vi "4_9.vi"() -> ()   [LabVIEW 2020]
panel:
  out "Output":string
  in  "Input":string
  out "substring":string
  out "Array":string[](array[string])
  in  "string":string
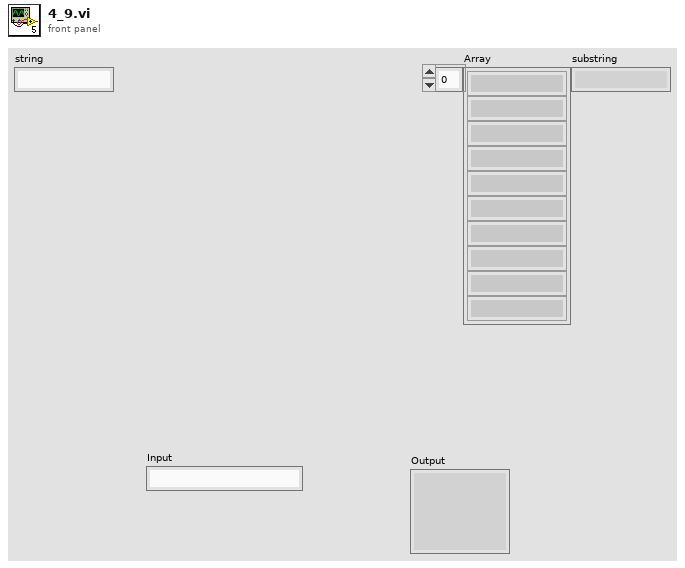
[diagram p1: front panel]
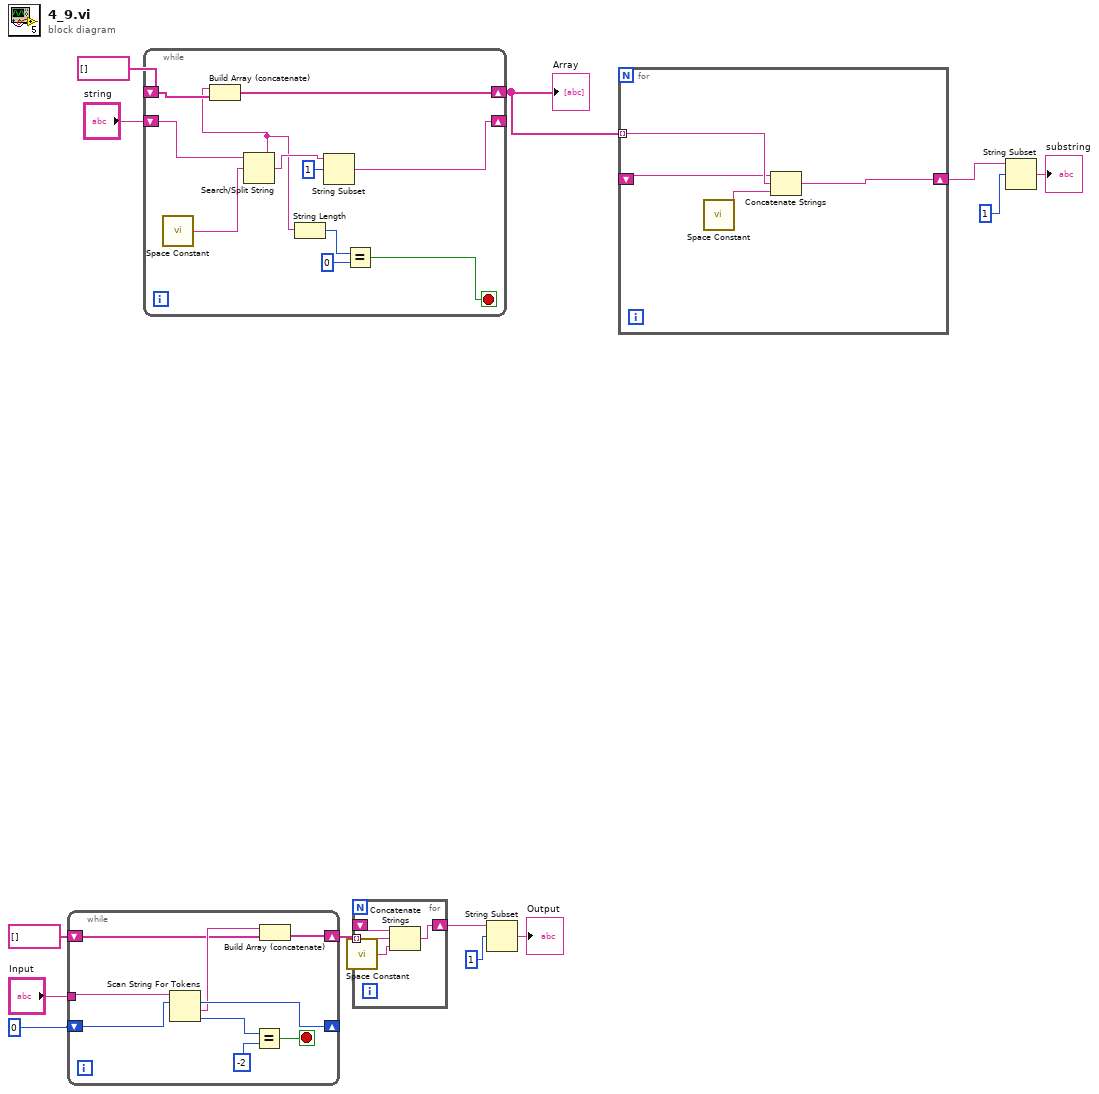
[diagram p0: block diagram]
diagram:
  n1 = while {
    tunnel: "Input" -> [w22]
    shift-right: [w18] -> w5
    shift-left: string[] [] -> [w14]
    shift-right: [w17] -> _
    shift-left: 0 ("offset past token") -> [w16]
    stop <- w19 stop-if-true
    n2 = Scan String For Tokens(8:w16, 9:w22) -> (0:w21:i32, 1:w15:string, 2:w17:i32)  [unwired: 4 in, 1 out]
    n3 = Equal?(x=w21, y=-2) -> (x = y?=w19:bool)
    n4 = Build Array (concatenate)(w15, w14) -> (w18:string[])
  }
  n5 = while {
    shift-right: [w29] -> _
    shift-left: "string" -> [w33]
    shift-right: [w28] -> w11
    shift-left: string[] [] -> [w24]
    stop <- w25 stop-if-true
    n6 = call <vilib>:"Space Constant.vi"() -> ("String"=w32:string)
    n7 = Search/Split String(string=w33, search string/char (-)=w32) -> (substring before match=w23:string, match + rest of string=w30:string)  [unwired: 1 in, 1 out]
    n8 = Build Array (concatenate)(w23, w24) -> (w28:string[])
    n9 = String Length(string=w23) -> (length=w27:i32)
    n10 = String Subset(string=w30, offset (0)=1) -> (substring=w29:string)  [unwired: 1 in]
    n11 = Equal?(x=w27, y=0) -> (x = y?=w25:bool)
  }
  "Array" <- w11
  n12 = for {
    tunnel: w5 -> [w37] mode=indexing
    shift-right: [w35] -> w4
    shift-left: _ -> [w36]
    n13 = call <vilib>:"Space Constant.vi"() -> ("String"=w34:string)
    n14 = Concatenate Strings(w36, w37, w34) -> (w35:string)
  }
  n15 = String Subset(string=w4, offset (0)=1) -> (substring=→"Output":string)  [unwired: 1 in]
  n16 = for {
    tunnel: w11 -> [w41] mode=indexing
    shift-right: [w40] -> w9
    shift-left: _ -> [w39]
    n17 = call <vilib>:"Space Constant.vi"() -> ("String"=w38:string)
    n18 = Concatenate Strings(w39, w41, w38) -> (w40:string)
  }
  n19 = String Subset(string=w9, offset (0)=1) -> (substring=→"substring":string)  [unwired: 1 in]
